vi "Launch IED Actor.vi"(8 "error in":errorcluster, 10 "Discovery Mode? (F)":bool, 11 "SCADA in":refnum<class "EMS.lvclass">) -> (0 "error out":errorcluster, 3 "SCADA out":refnum<class "EMS.lvclass">)   [LabVIEW 2018, in "EMS Core.lvlib" / "EMS.lvclass"]
uses:
  EMS.lvclass
  C:/Users/Administrator/Desktop/LabVIEW EMS/EMS Generic Actor/EMS Generic/EMS Generic.lvclass
  C:/Program Files (x86)/National Instruments/LabVIEW 2018/vi.lib/ActorFramework/Actor/Actor.lvclass
  IED Actors/IED Actor/IED/IED.lvclass
  EMS.lvclass/EMS.ctl
  <vilib>/ActorFramework/Actor/Actor.lvclass
  EMS Generic Actor/EMS Generic/EMS Generic.lvclass
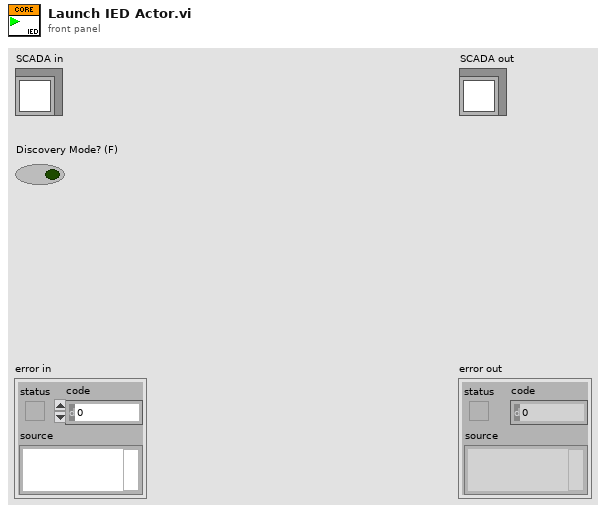
[diagram p1: front panel]
types:
  T1 = typedef "CSEISMIC DDS.lvlib/CSEISMIC DDS.lvclass/DeviceID.ctl" = string
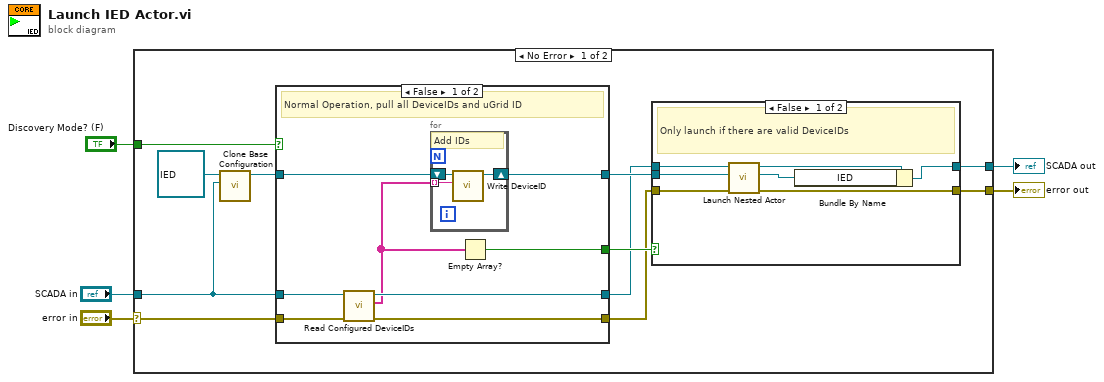
[diagram p0: block diagram]
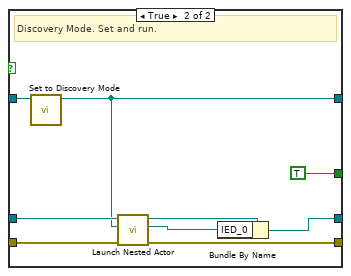
[diagram p2: hidden frame]
diagram:
  n1 = case shown="No Error" "error in" {
    selector: "error in" -> [w9 w47]
    tunnel: [w15 w47] -> w4
    tunnel: [w16 w46] -> w2
    tunnel: "SCADA in" -> [w7 w46]
    tunnel: "Discovery Mode? (F)" -> [w12 _]
    frame No Error {
      n2 = call-dynamic "Clone Base Configuration.vi"("Source Object"=w7, "Target Object in"=refnum<class "IED.lvclass"> refnum ("IED Actor.lvlib:IED.lvclass")) -> ("Target Object out"=w6:refnum<class "IED.lvclass">)  [unwired: 9 in]
      n3 = case shown="False" w12 {
        tunnel: [w24 w28] -> w14
        tunnel: w7 -> [w19 w33]
        tunnel: [w23 TRUE ("empty?")] -> w13
        tunnel: w6 -> [w22 w36]
        tunnel: w9 -> [w21 w30]
        tunnel: [w20 w29] -> w11
        tunnel: [w18 w31] -> w10
        frame False {
          # "Normal Operation, pull all DeviceIDs and uGrid ID"
          n4 = call "Read Configured DeviceIDs.vi"("error in"=w21, "EMS Generic in"=w19) -> ("error out"=w20:errorcluster, "DeviceIDs"=w17:T1[], "EMS Generic out"=w18:refnum<class "EMS.lvclass">)  [unwired: 7 in]
          n5 = for {
            shift-right: [w26] -> w24
            shift-left: w22 -> [w27]
            tunnel: w17 -> [w25] mode=indexing
            # "Add IDs"
            n6 = call-dynamic "Write DeviceID.vi"("DeviceID"=w25, "Device DDS Communications in"=w27) -> ("Device DDS Communications out"=w26:refnum<class "IED.lvclass">)  [unwired: 9 in]
          }
          n7 = Empty Array?(array=w17) -> (empty?=w23:bool)
        }
        frame True {
          # "Discovery Mode. Set and run."
          n8 = call "Set to Discovery Mode.vi"("IED in"=w36) -> ("IED out"=w28:refnum<class "IED.lvclass">)  [unwired: 10 in]
          n9 = call <vilib>:"Launch Nested Actor.vi"("error in (no error)"=w30, "Nested Actor"=w28, "Caller Actor in"=w33) -> ("error out"=w29:errorcluster, "Nested Actor's Enqueuer"=w34:refnum<class "Message Enqueuer.lvclass">, "Caller Actor out"=w32:refnum<class "EMS.lvclass">)  [unwired: 6 in]
          n10 = Bundle By Name(cluster=w32, "IED_0"=w34) -> (w31:refnum<class "EMS.lvclass">)
        }
      }
      n11 = case shown="False" w13 {
        tunnel: [w38 w45] -> w16
        tunnel: w11 -> [w42 w44]
        tunnel: [w41 w44] -> w15
        tunnel: w14 -> [w40 _]
        tunnel: w10 -> [w39 w45]
        frame False {
          # "Only launch if there are valid DeviceIDs"
          n12 = call <vilib>:"Launch Nested Actor.vi"("error in (no error)"=w42, "Nested Actor"=w40, "Caller Actor in"=w39) -> ("error out"=w41:errorcluster, "Nested Actor's Enqueuer"=w37:refnum<class "Message Enqueuer.lvclass">, "Caller Actor out"=w43:refnum<class "EMS.lvclass">)  [unwired: 6 in]
          n13 = Bundle By Name(cluster=w43, "IED"=w37) -> (w38:refnum<class "EMS.lvclass">)
        }
        frame True {
        }
      }
    }
    frame Error {
    }
  }
  "error out" <- w4
  "SCADA out" <- w2
